vi "Destroy.vi"(8 "error in (no error)":errorcluster, 11 "reference in":refnum<class "Console.lvclass">) -> (0 "error out":errorcluster, 3 "reference out":refnum<class "Console.lvclass">)   [LabVIEW 2018, in "Console.lvclass"]
uses:
  Console.lvclass
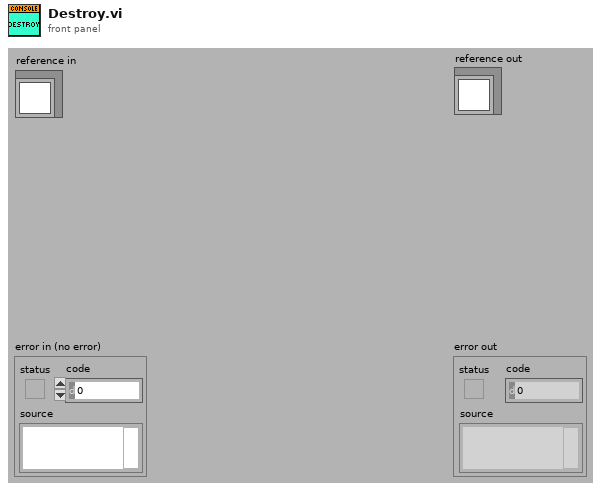
[diagram p1: front panel]
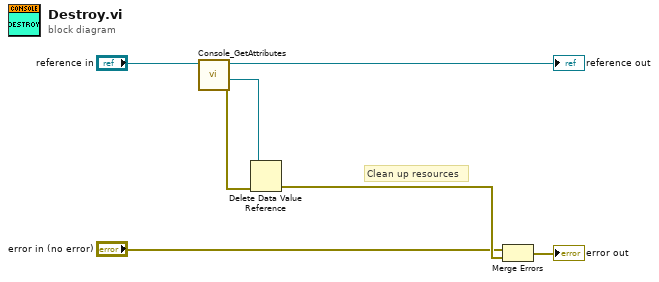
[diagram p0: block diagram]
diagram:
  # "Clean up resources"
  n1 = call "Console_GetAttributes.vi"("reference in"="reference in") -> ("error out"=w4:errorcluster, "DataRef"=w3:refnum<data-value>, "reference out"=→"reference out":refnum<class "Console.lvclass">)  [unwired: 7 in, 1 out]
  n2 = Delete Data Value Reference(data value reference=w3, error in=w4) -> (error out=w2:errorcluster)  [unwired: 1 out]
  n3 = Merge Errors("error in (no error)", w2) -> (→"error out":errorcluster)
